vi "Create.vi"(0 "Name":string, 5 "Cal Folder":path, 7 "Fs (Hz)":dbl=100000.0) -> (8 "State":refnum<class "State.lvclass">)   [LabVIEW 2020, in "State.lvclass"]
uses:
  State.lvclass
  Visual Stim VIs/Tosca-Grating.ctl
  Visual Stim VIs/Tosca-Grating Type.ctl
  State.lvclass/State.ctl
  Timeout/Timeout.lvclass
  epl-vi-lib/Signal Synthesis VIs/4th Generation/Classes/SignalManager/SignalManager.lvclass
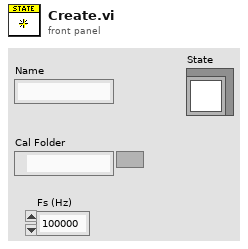
[diagram p1: front panel]
types:
  T1 = typedef "Tosca-Grating.ctl" = cluster{"Type":T2, "Orientation (deg)":dbl, "Spatial frequency (cpd)":dbl, "Velocity (Hz)":dbl, "Contrast":dbl, "Background intensity":dbl, "Duration (ms)":dbl, "Phase (cycles)":dbl}
  T2 = typedef "Tosca-Grating Type.ctl" = enum16{"OFF", "Square", "Sine"}
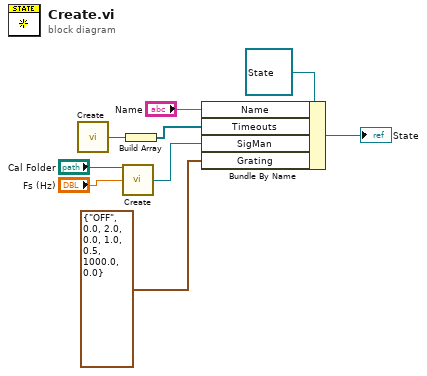
[diagram p0: block diagram]
diagram:
  n1 = call "Create.vi"() -> ("Timeout"=w6:refnum<class "Timeout.lvclass">)  [unwired: 15 in]
  n2 = call "Create.vi"("Cal Folder"="Cal Folder", "Fs (Hz)"="Fs (Hz)") -> ("SigMan"=w3:refnum<class "SignalManager.lvclass">)  [unwired: 13 in]
  n3 = Build Array(w6) -> (w5:refnum<class "Timeout.lvclass">[])
  n4 = Bundle By Name(cluster=refnum<class "State.lvclass"> refnum ("State"), "Name"="Name", "Timeouts"=w5, "SigMan"=w3, "Grating"=T1 {"Type"=enum."OFF", "Orientation (deg)"=0.0, "Spatial frequency (cpd)"=2.0, "Velocity (Hz)"=0.0, "Contrast"=1.0, "Background intensity"=0.5, "Duration (ms)"=1000.0, "Phase (cycles)"=0.0} ("Serialized.Grating")) -> (→"State":refnum<class "State.lvclass">)
